vi "Set speed.vi"(0 "VRN IN":refnum<visa-resource-name>, 1 "Bool Refnum":refnum<vi>, 11 "error IN":errorcluster) -> (4 "VRN OUT":refnum<visa-resource-name>, 8 "OK Done":bool, 15 "error out":errorcluster)   [LabVIEW 2019]
panel:
  in  "Vitesse":dbl=1.5 caption="Deg/sec" min=0.0 max=1.5 step=0.1 format="%.1f"
  in  "OK":bool
  in  "Été":bool caption="Deg/sec"
  in  "Hiver":bool caption="Deg/sec"
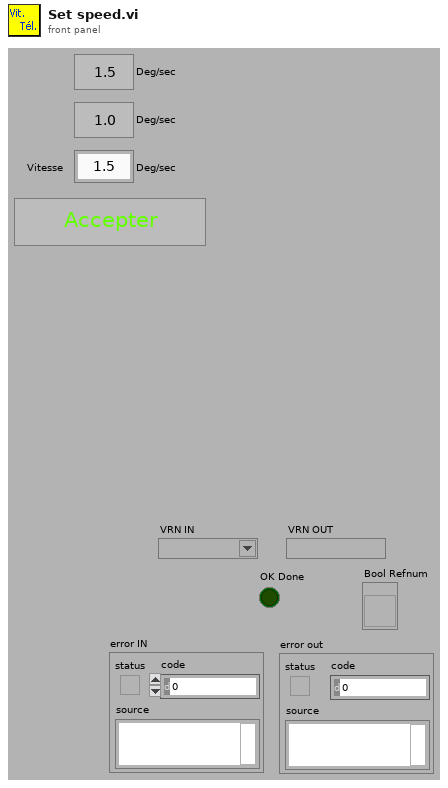
[diagram p1: front panel]
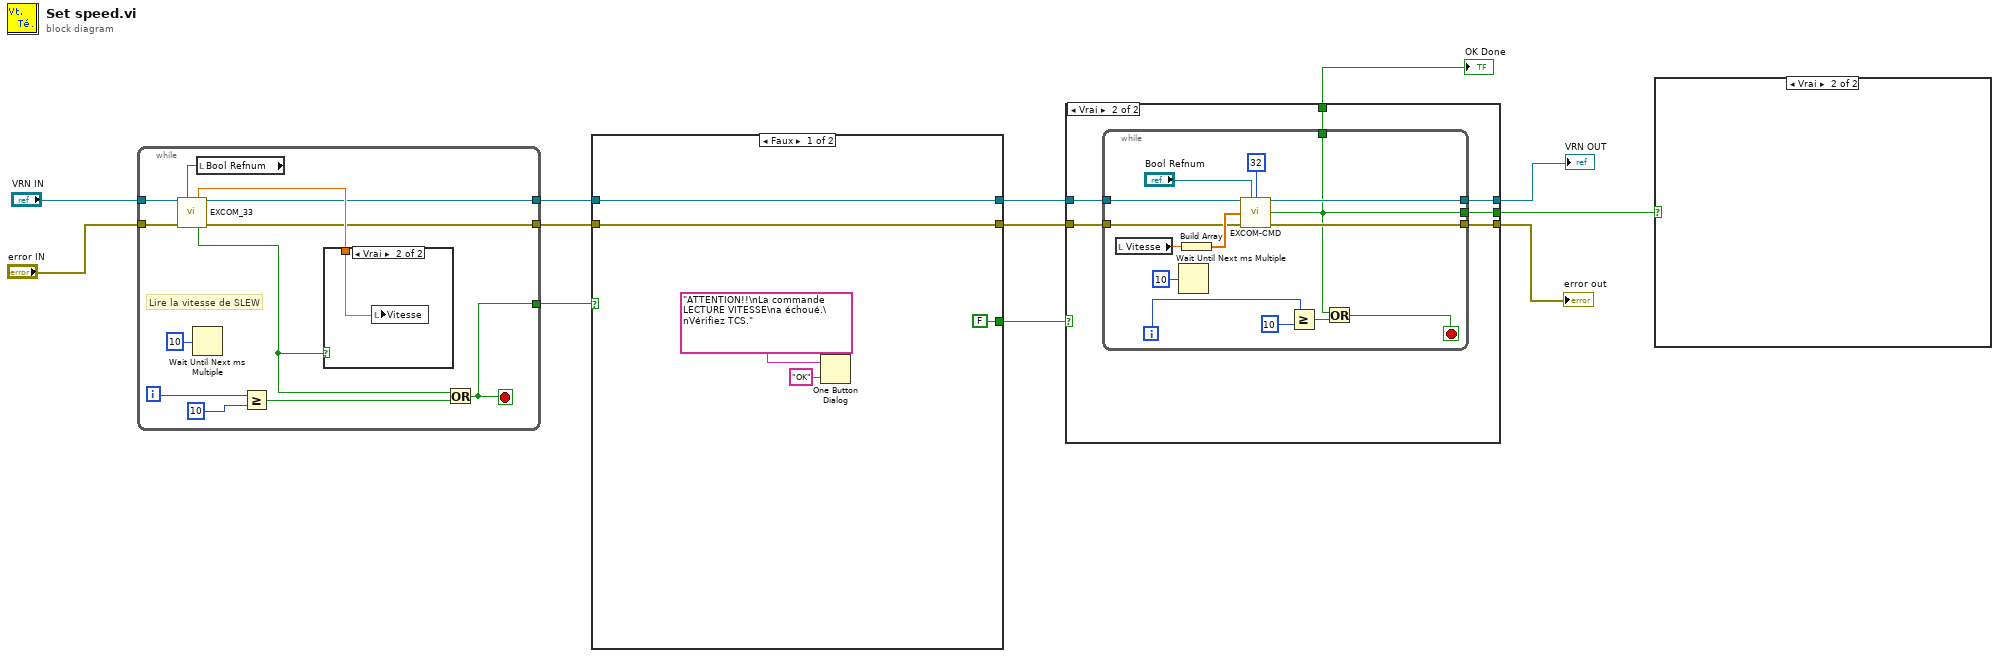
[diagram p0: block diagram]
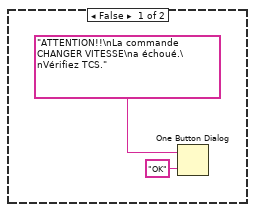
[diagram p2: hidden frame]
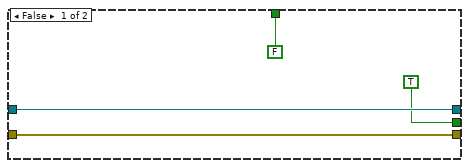
[diagram p3: hidden frame]
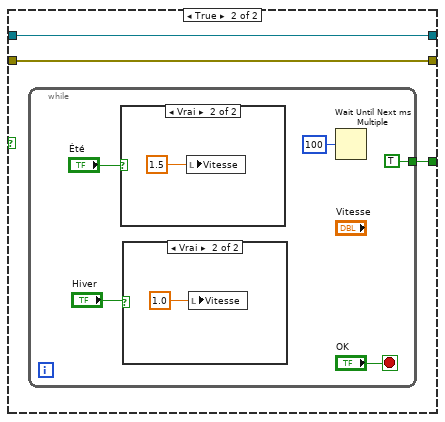
[diagram p4: hidden frame]
diagram:
  n1 = while {
    tunnel: "VRN IN" -> [w20]
    tunnel: "error IN" -> [w17]
    tunnel: [w16] -> w7
    tunnel: [w15] -> w8
    tunnel: [w14] -> w10
    i -> [w23]
    stop <- w14 stop-if-true
    # "Lire la vitesse de SLEW"
    n2 = Wait Until Next ms Multiple(millisecond multiple=u32 10 ("n millisecondes")) -> ()  [unwired: 1 out]
    n3 = local read "Bool Refnum"() -> (w13:refnum<vi>)
    n4 = call "EXCOM_33.vi"("VISA resource name"=w20, "Bool Refnum"=w13, "Error IN"=w17) -> ("Vtel"=w18:dbl, "VISA resource name dup"=w15:refnum<visa-resource-name>, "OK Done"=w19:bool, "error out"=w16:errorcluster)  [unwired: 9 in]
    n5 = Greater Or Equal?(x=w23, y=10) -> (x >= y?=w21:bool)
    n6 = case shown="Vrai" w19 {
      tunnel: w18 -> [_ w25]
      frame False {
      }
      frame True {
        n7 = local write "Vitesse"(w25) -> ()
      }
    }
    n8 = Or(x=w19, y=w21) -> (x .or. y?=w14:bool)
  }
  n9 = case shown="Faux" w10 {
    tunnel: [FALSE ("OK") w33] -> w9
    tunnel: [w27 w32] -> w6
    tunnel: w8 -> [w27 w32]
    tunnel: [w26 w31] -> w5
    tunnel: w7 -> [w26 w31]
    frame False {
      n10 = One Button Dialog(message="ATTENTION!!\nLa commande LECTURE VITESSE\na échoué.\nVérifiez TCS.", button name ("OK")="OK" ("nom du bouton (\"OK\")")) -> ()  [unwired: 1 out]
    }
    frame True {
      n11 = while {
        tunnel: [TRUE ("OK")] -> w33
        stop <- "OK" stop-if-true
        n12 = case shown="Vrai" "Été" {
          frame False {
          }
          frame True {
            n13 = local write "Vitesse"(1.5) -> ()
          }
        }
        n14 = case shown="Vrai" "Hiver" {
          frame False {
          }
          frame True {
            n15 = local write "Vitesse"(1.0) -> ()
          }
        }
        n16 = Wait Until Next ms Multiple(millisecond multiple=u32 100 ("n millisecondes")) -> ()  [unwired: 1 out]
      }
    }
  }
  n17 = case shown="Vrai" w9 {
    tunnel: w6 -> [w44 w50]
    tunnel: w5 -> [w43 w49]
    tunnel: [w44 w48] -> w2
    tunnel: [w43 w47] -> w3
    tunnel: [TRUE ("OK Done") w46] -> w4
    tunnel: [FALSE ("OK Done") w45] -> w1
    frame False {
    }
    frame True {
      n18 = while {
        tunnel: w50 -> [w56]
        tunnel: w49 -> [w55]
        tunnel: [w54] -> w48
        tunnel: [w53] -> w47
        tunnel: [w52] -> w46
        tunnel: [w52] -> w45
        i -> [w63]
        stop <- w60 stop-if-true
        n19 = local read "Vitesse"() -> (w58:dbl)
        n20 = Wait Until Next ms Multiple(millisecond multiple=u32 10 ("n millisecondes")) -> ()  [unwired: 1 out]
        n21 = Build Array(w58) -> (w59:dbl[])
        n22 = call "EXCOM-CMD.vi"("VRN IN"=w56, "Bool Refnum"="Bool Refnum", "Commande #"=32 ("NombredArguments"), "Args"=w59, "Error IN"=w55) -> ("VRN OUT"=w54:refnum<visa-resource-name>, "OK Done"=w52:bool, "Error OUT"=w53:errorcluster)  [unwired: 8 in]
        n23 = Greater Or Equal?(x=w63, y=10) -> (x >= y?=w64:bool)
        n24 = Or(x=w52, y=w64) -> (x .or. y?=w60:bool)
      }
    }
  }
  "VRN OUT" <- w2
  "error out" <- w3
  "OK Done" <- w1
  n25 = case shown="Vrai" w4 {
    frame False {
      n26 = One Button Dialog(message="ATTENTION!!\nLa commande CHANGER VITESSE\na échoué.\nVérifiez TCS.", button name ("OK")="OK" ("nom du bouton (\"OK\")")) -> ()  [unwired: 1 out]
    }
    frame True {
    }
  }
